vi "DAQmx Create Channel (AI-Torque-Bridge-Table).vi"(0 "task in":refnum<k21>, 1 "maximum value":dbl=100.0 format="%0.2f", 2 "minimum value":dbl=-100.0 format="%0.2f", 3 "bridge information":T1={"bridge configuration"=10182, "voltage excitation source"=10200, "voltage excitation value"=2.5, "nominal bridge resistance"=350.0} {"voltage excitation source" items=["Internal"=10200, "External"=10167]; "bridge configuration" items=["Full Bridge"=10182, "Half Bridge"=10187, "Quarter Bridge"=10270]}, 5 "physical channels":tag, 7 "name to assign":string, 9 "units":i32(ring)=15883 items=["Nm"=15881, "oz-in"=15882, "lb-in"=15883, "lb-ft"=15884, "From Custom Scale"=10065], 11 "error in":errorcluster, 12 "custom scale name":tag, 14 "scaling information":T2={"electrical values"=[-2.0, 0.0, 2.0], "electrical units"=15897, "physical values"=[-100.0, 0.0, 100.0], "physical units"=15883} {"electrical units" items=["Volts/Volt"=15896, "mVolts/Volt"=15897]; "physical units" items=["Nm"=15881, "oz-in"=15882, "lb-in"=15883, "lb-ft"=15884]}) -> (4 "task out":refnum<k21>, 15 "error out":errorcluster)   [LabVIEW 2013]
doc: "Creates channel(s) that use a Wheatstone bridge to measure torque. Use this instance with sensors whose specifications provide a table of electrical values and the corresponding physical values. When you use this scaling type, NI-DAQmx performs linear scaling between each pair of electrical and physical values. The input limits specified with <B>minimum value</B> and <B>maximum value</B> must fall within the smallest and largest physical values. For any data outside those endpoints, NI-DAQmx coerces that data to the endpoints."
uses:
  nilvaiu.dll
panel:
  # "input limits"
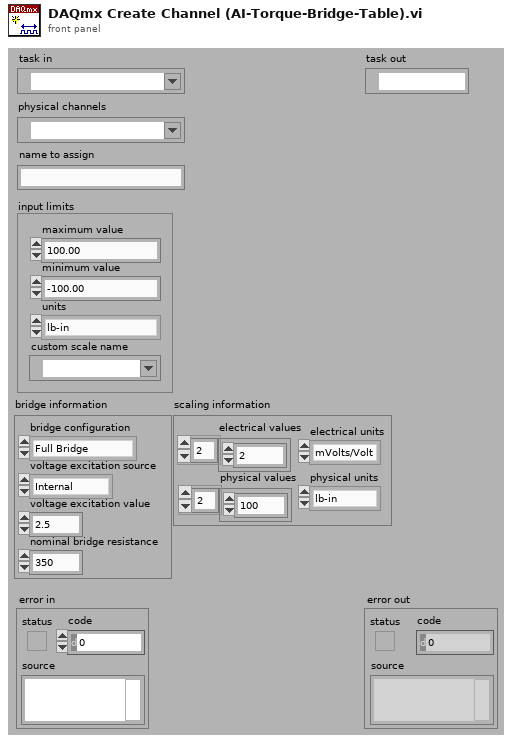
[diagram p1: front panel]
types:
  T1 = cluster{"bridge configuration":i32, "voltage excitation source":i32, "voltage excitation value":dbl, "nominal bridge resistance":dbl}
  T2 = cluster{"electrical values":dbl[], "electrical units":i32, "physical values":dbl[], "physical units":i32}
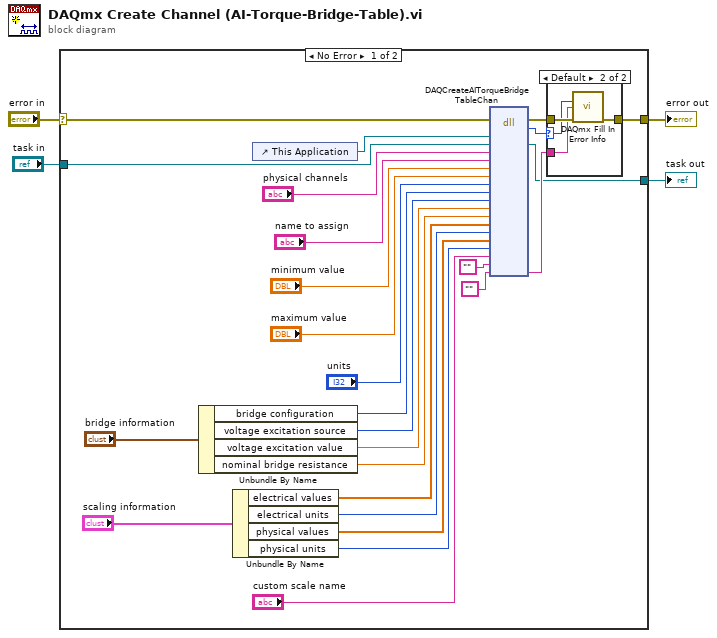
[diagram p0: block diagram]
diagram:
  n1 = case shown="No Error" "error in" {
    selector: "error in" -> [w8 w36]
    tunnel: "task in" -> [w10 w37]
    tunnel: [w9 w37] -> w3
    tunnel: [w7 w36] -> w1
    frame No Error {
      n2 = Unbundle By Name("bridge information") -> ("bridge configuration"=w24:i32, "voltage excitation source"=w25:i32, "voltage excitation value"=w26:dbl, "nominal bridge resistance"=w27:dbl)
      n3 = Unbundle By Name("scaling information") -> ("electrical values"=w20:dbl[], "electrical units"=w21:i32, "physical values"=w22:dbl[], "physical units"=w23:i32)
      n4 = control-ref of="This Application"() -> (w13:refnum<vi>)
      n5 = dll-call lib="nilvaiu.*" fn="DAQCreateAITorqueBridgeTableChan"(error in=w8, "lvAppRef"=w13, "refObjPtr"=w10, "physicalChannelName"="physical channels", "channelNameIn"="name to assign", "minVal"="minimum value", "maxVal"="maximum value", "units"="units", "bridgeConfig"=w24, "voltageExcitSource"=w25, "voltageExcitVal"=w26, "nominalBridgeResistance"=w27, "electricalValues"=w20, "electricalUnits"=w21, "physicalValues"=w22, "physicalUnits"=w23, "customScaleName"="custom scale name", "channelNamesOut"="", "extendedErrorInfo"="") -> (error out=w30:errorcluster, "return type"=w29:i32, "refObjPtr"=w9:refnum<k21>, "extendedErrorInfo"=w28:string)  [unwired: 18 in, 1 out]
      n6 = case shown="Default" w29 {
        selector: w29 -> [_ w33]
        tunnel: w30 -> [w31 w35]
        tunnel: [w31 w34] -> w7
        tunnel: w28 -> [_ w32]
        frame 0 {
        }
        frame Default {
          n7 = call "DAQmx Fill In Error Info.vi"("status code"=w33, "extended error info"=w32, "error in"=w35) -> ("error out"=w34:errorcluster)  [unwired: 1 in, 11 out]
        }
      }
    }
    frame Error {
    }
  }
  "task out" <- w3
  "error out" <- w1
